vi "MuC_Read_Values.vi"(0 "VISA resource name":refnum<visa-resource-name>, 1 "Nreads":i32, 2 "Delay (ms)":u32=4000 min=4000 max=20000, 3 "Read Type":enum16{"SMPL", "DC", "AC"}(ring), 4 "error in (no error)":errorcluster) -> (5 "VISA resource name 2":refnum<visa-resource-name>, 6 "Buffer Data":string[](array[string]), 7 "error out":errorcluster)   [LabVIEW 2019]
doc: "Send a command to a MicroController telling it to read a voltage\nThis VI performs multiple reads and formats the data in the read buffer to output numerical values. \nMinimum delay between read commands is 1000 ms, otherwise an error is thrown \n\nR. Sheehan 28 - 10 - 2020"
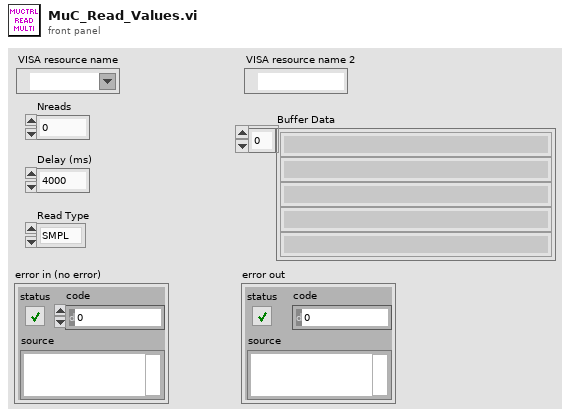
[diagram p1: front panel]
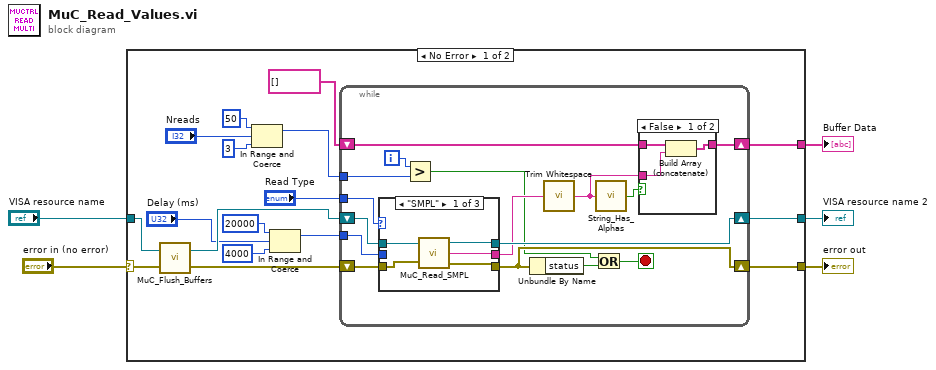
[diagram p0: block diagram]
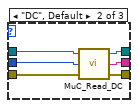
[diagram p2: hidden frame]
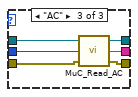
[diagram p3: hidden frame]
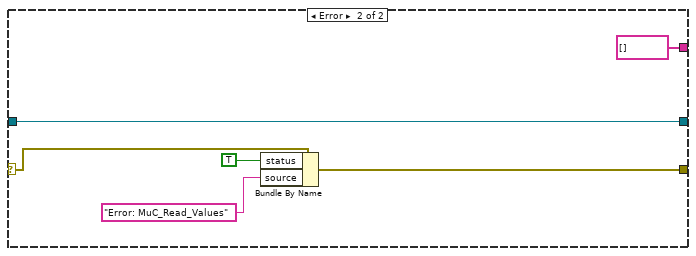
[diagram p5: hidden frame]
diagram:
  n1 = case shown="No Error" "error in (no error)" {
    selector: "error in (no error)" -> [w18 w65]
    tunnel: [w16 w64] -> w4
    tunnel: "VISA resource name" -> [w19 w61]
    tunnel: [w17 w61] -> w2
    tunnel: [w15 string[] []] -> w1
    frame No Error {
      n2 = call "MuC_Flush_Buffers.vi"("error in (no error)"=w18, "VISA resource name"=w19) -> ("error out"=w20:errorcluster, "VISA resource name 2"=w21:refnum<visa-resource-name>)
      n3 = In Range and Coerce(upper limit=50, x="Nreads", lower limit=3) -> (coerced(x)=w11:i32)  [unwired: 1 out]
      n4 = In Range and Coerce(upper limit=u32 20000, x="Delay (ms)", lower limit=u32 4000) -> (coerced(x)=w6:u32)  [unwired: 1 out]
      n5 = while {
        shift-right: [w33] -> w17
        shift-left: w21 -> [w35]
        shift-right: [w27] -> w16
        shift-left: w20 -> [w34]
        shift-right: [w36] -> w15
        shift-left: string[] [] -> [w37]
        tunnel: w11 -> [w31]
        tunnel: "Read Type" -> [w28]
        tunnel: w6 -> [w23]
        i -> [w38]
        stop <- w26 stop-if-true
        n6 = case shown="\"SMPL\"" w28 {
          tunnel: w35 -> [w41 w47 w55]
          tunnel: w34 -> [w43 w48 w54]
          tunnel: [w40 w46 w53] -> w33
          tunnel: [w42 w49 w52] -> w27
          tunnel: [w39 w45 w51] -> w32
          tunnel: w23 -> [_ w44 w50]
          frame "SMPL" {
            n7 = call "MuC_Read_SMPL.vi"("VISA resource name"=w41, "error in (no error)"=w43) -> ("VISA resource name 2"=w40:refnum<visa-resource-name>, "Cmd"=w39:string, "error out"=w42:errorcluster)
          }
          frame "DC", Default {
            n8 = call "MuC_Read_DC.vi"("error in (no error)"=w48, "Delay / ms"=w44, "VISA resource name"=w47) -> ("error out"=w49:errorcluster, "Cmd"=w45:string, "VISA resource name 2"=w46:refnum<visa-resource-name>)
          }
          frame "AC" {
            n9 = call "MuC_Read_AC.vi"("error in (no error)"=w54, "Delay / ms"=w50, "VISA resource name"=w55) -> ("error out"=w52:errorcluster, "Cmd"=w51:string, "VISA resource name 2"=w53:refnum<visa-resource-name>)
          }
        }
        n10 = Greater?(x=w38, y=w31) -> (0:w24:bool)
        n11 = Unbundle By Name(w27) -> ("status"=w25:bool)
        n12 = call <vilib>:"Trim Whitespace.vi"("string"=w32) -> ("trimmed string"=w30:string)  [unwired: 1 in]
        n13 = Or(x=w24, y=w25) -> (x .or. y?=w26:bool)
        n14 = call "String_Has_Alphas.vi"("input string"=w30) -> ("String Has Alphas"=w29:bool)
        n15 = case shown="False" w29 {
          tunnel: w37 -> [w58 w59]
          tunnel: [w57 w59] -> w36
          tunnel: w30 -> [w56 _]
          frame False {
            n16 = Build Array (concatenate)(w58, w56) -> (w57:string[])
          }
          frame True {
          }
        }
      }
    }
    frame Error {
      n17 = Bundle By Name(cluster=w65, "status"=TRUE, "source"="Error: MuC_Read_Values") -> (w64:errorcluster)
    }
  }
  "error out" <- w4
  "VISA resource name 2" <- w2
  "Buffer Data" <- w1
